vi "用户读写.vi"(7 "Enum":T1(ring)=enum."read", 9 "值":string, 10 "键":string, 11 "字段":string) -> (1 "字段名称":string[](array[string]), 2 "键名称":string[](array[string]), 3 "读取到的值":string)   [LabVIEW 2020]
uses:
  <vilib>/Utility/config.llb/Write Key (String).vi
  <vilib>/Utility/config.llb/Read Key (String).vi
  <vilib>/Utility/config.llb/NI_LVConfig.lvlib
panel:
  out "error out":errorcluster
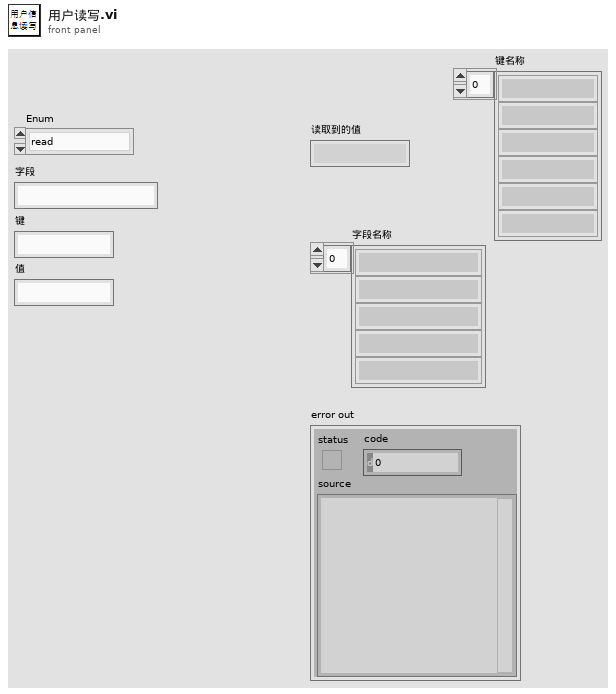
[diagram p1: front panel]
types:
  T1 = enum16{"write", "read", "read_key", "read_section"}
  T2 = typedef "NI_LVConfig.lvlib/Config Data RefNum.ctl" = refnum<k1>
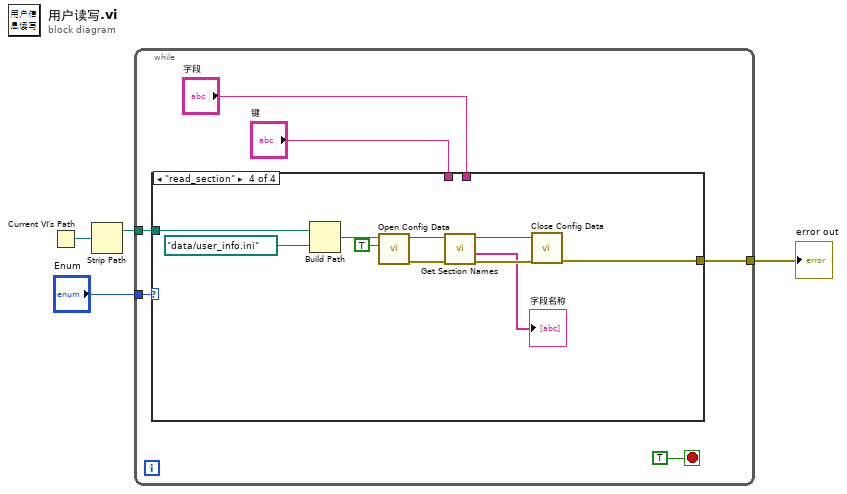
[diagram p0: block diagram]
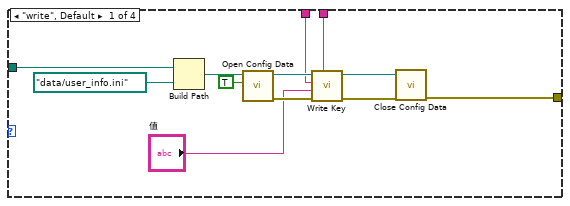
[diagram p2: hidden frame]
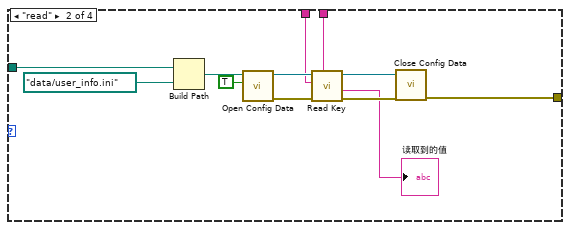
[diagram p3: hidden frame]
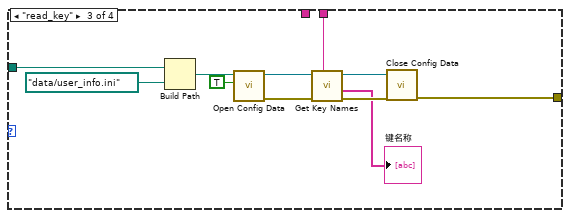
[diagram p4: hidden frame]
diagram:
  n1 = Current VI's Path() -> (path=w1:path)
  n2 = Strip Path(path=w1) -> (stripped path=w2:path)  [unwired: 1 out]
  n3 = while {
    tunnel: "Enum" -> [w9]
    tunnel: [w6] -> w3
    tunnel: w2 -> [w5]
    stop <- TRUE stop-if-true
    n4 = case shown="\"read_section\"" w9 {
      tunnel: "字段" -> [w15 w26 w37 _]
      tunnel: "键" -> [w14 w25 _ _]
      tunnel: [w12 w27 w38 w47] -> w6
      tunnel: w5 -> [w11 w23 w35 w46]
      frame "write", Default {
        n5 = Build Path(base path=w11, name or relative path=path "data/user_info.ini") -> (appended path=w21:path)
        n6 = call <vilib>:"Open Config Data.vi"("create file if necessary (T)"=TRUE, "configuration file path"=w21) -> ("error out"=w18:errorcluster, "refnum"=w19:T2)  [unwired: 7 in, 1 out]
        n7 = call-poly <vilib>:"Write Key.vi"("section"=w15, "error in (no error)"=w18, "value"="值", "key"=w14, "refnum"=w19) -> ("error out"=w17:errorcluster, "refnum out"=w16:T2)  [unwired: 4 in, 1 out]
        n8 = call <vilib>:"Close Config Data.vi"("error in (no error)"=w17, "refnum"=w16) -> ("error out"=w12:errorcluster)  [unwired: 8 in, 1 out]
      }
      frame "read" {
        n9 = Build Path(base path=w23, name or relative path=path "data/user_info.ini") -> (appended path=w30:path)
        n10 = call <vilib>:"Open Config Data.vi"("create file if necessary (T)"=TRUE, "configuration file path"=w30) -> ("error out"=w32:errorcluster, "refnum"=w31:T2)  [unwired: 7 in, 1 out]
        n11 = call-poly <vilib>:"Read Key.vi"("section"=w26, "error in (no error)"=w32, "key"=w25, "refnum"=w31) -> ("error out"=w33:errorcluster, "value"=→"读取到的值":string, "refnum out"=w34:T2)  [unwired: 4 in, 1 out]
        n12 = call <vilib>:"Close Config Data.vi"("error in (no error)"=w33, "refnum"=w34) -> ("error out"=w27:errorcluster)  [unwired: 8 in, 1 out]
      }
      frame "read_key" {
        n13 = Build Path(base path=w35, name or relative path=path "data/user_info.ini") -> (appended path=w41:path)
        n14 = call <vilib>:"Open Config Data.vi"("create file if necessary (T)"=TRUE, "configuration file path"=w41) -> ("error out"=w43:errorcluster, "refnum"=w42:T2)  [unwired: 7 in, 1 out]
        n15 = call <vilib>:"Get Key Names.vi"("section"=w37, "error in (no error)"=w43, "refnum"=w42) -> ("error out"=w44:errorcluster, "key names"=→"键名称":string[], "refnum out"=w45:T2)  [unwired: 5 in, 1 out]
        n16 = call <vilib>:"Close Config Data.vi"("error in (no error)"=w44, "refnum"=w45) -> ("error out"=w38:errorcluster)  [unwired: 8 in, 1 out]
      }
      frame "read_section" {
        n17 = Build Path(base path=w46, name or relative path=path "data/user_info.ini") -> (appended path=w51:path)
        n18 = call <vilib>:"Open Config Data.vi"("create file if necessary (T)"=TRUE, "configuration file path"=w51) -> ("error out"=w53:errorcluster, "refnum"=w52:T2)  [unwired: 7 in, 1 out]
        n19 = call <vilib>:"Get Section Names.vi"("error in (no error)"=w53, "refnum"=w52) -> ("error out"=w54:errorcluster, "section names"=→"字段名称":string[], "refnum out"=w55:T2)  [unwired: 7 in]
        n20 = call <vilib>:"Close Config Data.vi"("error in (no error)"=w54, "refnum"=w55) -> ("error out"=w47:errorcluster)  [unwired: 8 in, 1 out]
      }
    }
  }
  "error out" <- w3
